vi "Match value to time constant.vi"(1 "Tau":T1 items=["10 us", "30 us", "100 us", "300 us", "1 ms", "3 ms", "10 ms", "30 ms", "100 ms", "300 ms", "1 s", "3 s", "10 s", "30 s", "100 s", "300 s", "1 ks", "3 ks", "10 ks", "30 ks"]) -> (0 "time constant":dbl[unit])   [LabVIEW 2023, in "SR830.lvlib"]
doc: "Takes an integer input (the value returned by the lock-in) and matches it to its corresponding time constant."
uses:
  SR830.lvlib
  Tau.ctl
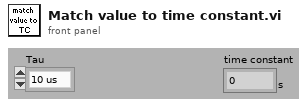
[diagram p1: front panel]
types:
  T1 = typedef "SR830.lvlib/Tau.ctl" = u16
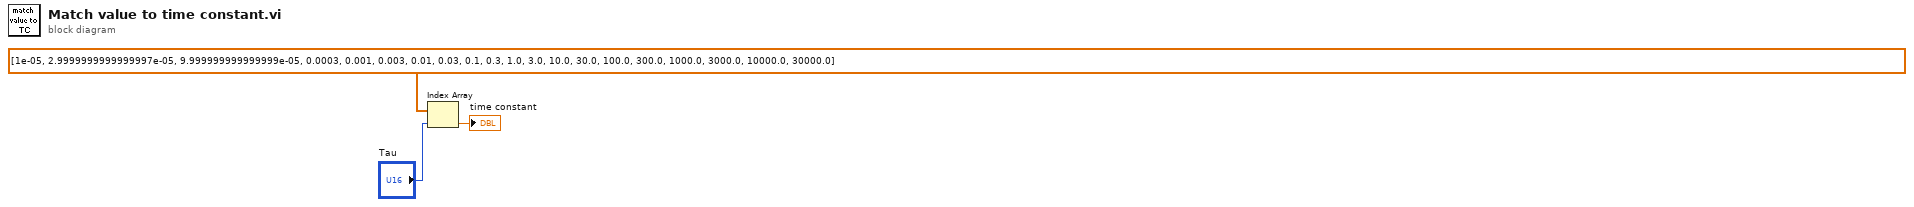
[diagram p0: block diagram]
diagram:
  n1 = Index Array(array=dbl[unit][] [1e-05, 2.9999999999999997e-05, 9.999999999999999e-05, 0.0003, 0.001, 0.003, 0.01, 0.03, 0.1, 0.3, 1.0, 3.0, 10.0, 30.0, 100.0, 300.0, 1000.0, 3000.0, 10000.0, 30000.0] ("Array"), index="Tau") -> (element=→"time constant":dbl[unit])
